vi "roboRIO v1.0 Unreserve RSL.vi"(7 "Allow multiple opens?":bool, 8 "error in (no error)":errorcluster, 10 "RSL Channel List":T1) -> (0 "error out":errorcluster)   [LabVIEW 2021]
uses:
  <vilib>/myRIO/Common/Instrument Driver Framework/roboRIO v1.0/RSL/typedefs/RSL Channels List.ctl
  <vilib>/myRIO/Common/Instrument Driver Framework/roboRIO v1.0/RSL/typedefs/RSL Channels Enum.ctl
  <vilib>/myRIO/Common/Instrument Driver Framework/roboRIO v1.0/Resource Manager/vis/roboRIO v1.0 Unreserve Channel.vi
  <vilib>/myRIO/Common/Instrument Driver Framework/roboRIO v1.0/Resource Manager/vis/roboRIO v1.0 Build Mutex Name.vi
  <vilib>/myRIO/Common/Instrument Driver Framework/Utilities/vis/Configuration Manager.vi
  <vilib>/myRIO/Common/Instrument Driver Framework/Utilities/vis/IO Manager.vi
  <vilib>/Utility/error.llb/Error Cluster From Error Code.vi
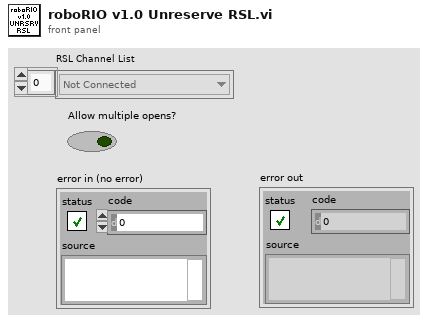
[diagram p1: front panel]
types:
  T1 = typedef "RSL Channels List.ctl" = T2[]
  T2 = typedef "RSL Channels Enum.ctl" = enum16{"Not Connected", "RSL/RSL0"}
  T3 = typedef "roboRIO v1.0 Channel Reservation List.ctl" = T4[]
  T4 = typedef "roboRIO v1.0 Channel Reservation Info.ctl" = cluster{"Channel Name":string, "Connector":T5, "Mutex ID":i32}
  T5 = typedef "roboRIO v1.0 Connector List.ctl" = enum32{"None", "ConnectorB", "ConnectorI2C", "ConnectorDIO", "ConnectorRSL", "ConnectorRELAY", "ConnectorAI", "ConnectorPWM", "ConnectorSPI"}
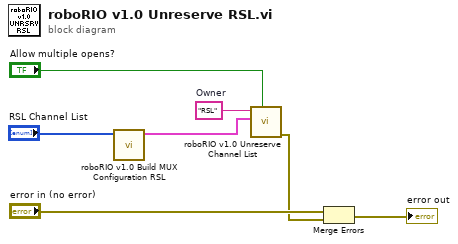
[diagram p0: block diagram]
diagram:
  w1 = "RSL"  # Owner
  n1 = call <vilib>:"roboRIO v1.0 Build MUX Configuration RSL.vi"("RSL Channel List"="RSL Channel List") -> ("Channel Reservation List"=w3:T3)  [unwired: 10 in]
  n2 = call <vilib>:"roboRIO v1.0 Unreserve Channel List.vi"("Allow multiple opens?"="Allow multiple opens?", "Channel Reservation List"=w3, "Owner"=w1) -> ("error out"=w2:errorcluster)  [unwired: 8 in]
  n3 = Merge Errors("error in (no error)", w2) -> (→"error out":errorcluster)
